vi "Disable Button.vi"(10 "Disabled":T1(ring)=enum."Disabled and Grayed Out", 11 "ctrl ref in":refnum<vi>) -> ()   [LabVIEW 2020, in "FrameEditor.lvlib"]
uses:
  FrameEditor.lvlib
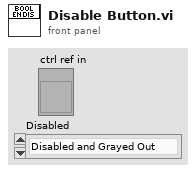
[diagram p1: front panel]
types:
  T1 = enum8{"Enabled", "Disabled", "Disabled and Grayed Out"}
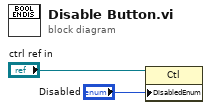
[diagram p0: block diagram]
diagram:
  n1 = property class="Ctl"(reference="ctrl ref in", "DisabledEnum"="Disabled") -> ()  [unwired: 1 in, 2 out]
